vi "Unload Theme.vi"(8 "Error In":errorcluster, 11 "ini Theme in":refnum<class "ini Theme.lvclass">) -> (0 "Error Out":errorcluster, 3 "ini Theme out":refnum<class "ini Theme.lvclass">)   [LabVIEW 2021, in "Appearance Actor.lvlib" / "ini Theme.lvclass"]
uses:
  ini Theme.lvclass
  C:/Users/Thomas/Documents/Projects/TemplateVIEW/Sources/Appearance Actor/Theme Classes/Generic Theme/Generic Theme.lvclass
  <vilib>/Utility/config.llb/Config Data RefNum.ctl
  Generic Theme/Generic Theme.lvclass/Generic Theme.ctl
  ini Theme.lvclass/ini Theme.ctl
  <vilib>/Utility/config.llb/NI_LVConfig.lvlib
  Generic Theme/Generic Theme.lvclass
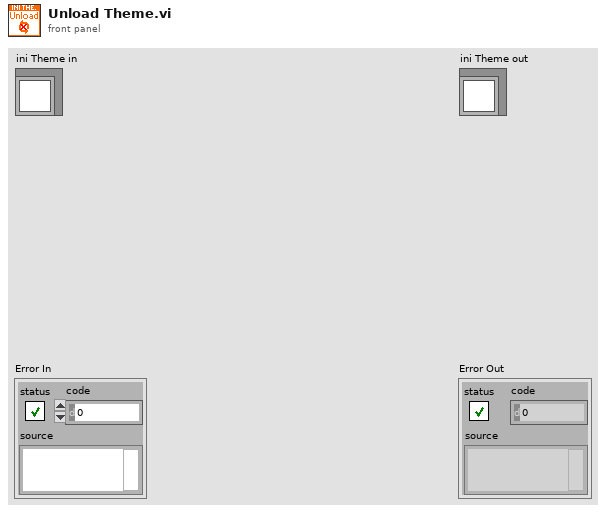
[diagram p1: front panel]
types:
  T1 = typedef "NI_LVConfig.lvlib/Config Data RefNum.ctl" = refnum<k1>
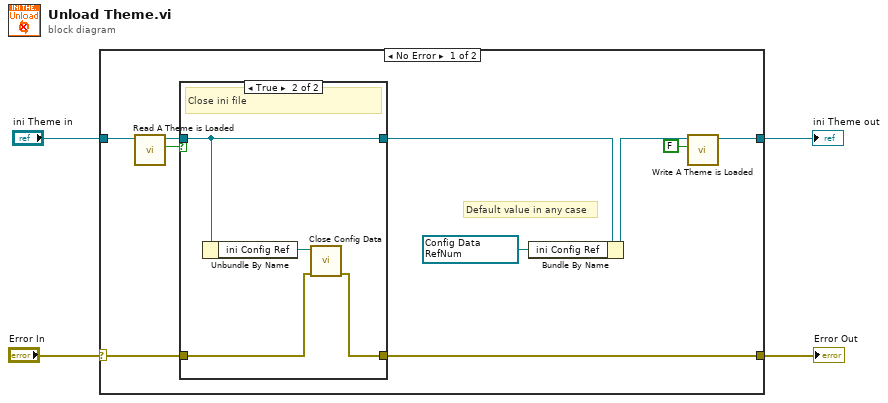
[diagram p0: block diagram]
diagram:
  n1 = case shown="No Error" "Error In" {
    selector: "Error In" -> [w14 w22]
    tunnel: [w13 w22] -> w3
    tunnel: "ini Theme in" -> [w10 w21]
    tunnel: [w6 w21] -> w1
    frame No Error {
      w11 = T1 refnum items=["config data"] ("Theme Data.ini Config Ref")
      # "Default value in any case"
      n2 = call "Read A Theme is Loaded.vi"("Generic Theme in"=w10) -> ("A Theme is Loaded"=w8:bool, "Generic Theme out"=w9:refnum<class "ini Theme.lvclass">)  [unwired: 8 in, 1 out]
      n3 = case shown="True" w8 {
        tunnel: w14 -> [w15 w19]
        tunnel: [w15 w18] -> w13
        tunnel: w9 -> [w16 w17]
        tunnel: [w16 w17] -> w7
        frame False {
          # "No theme do nothing"
        }
        frame True {
          # "Close ini file"
          n4 = Unbundle By Name(w17) -> ("ini Config Ref"=w20:T1)
          n5 = call <vilib>:"Close Config Data.vi"("error in (no error)"=w19, "refnum"=w20) -> ("error out"=w18:errorcluster)  [unwired: 8 in, 1 out]
        }
      }
      n6 = Bundle By Name(cluster=w7, "ini Config Ref"=w11) -> (w12:refnum<class "ini Theme.lvclass">)
      n7 = call "Write A Theme is Loaded.vi"("A Theme is Loaded"=FALSE, "Generic Theme in"=w12) -> ("Generic Theme out"=w6:refnum<class "ini Theme.lvclass">)  [unwired: 8 in, 1 out]
    }
    frame Error {
    }
  }
  "Error Out" <- w3
  "ini Theme out" <- w1
